vi "Simple TCP 채팅- Server.vi"() -> ()   [LabVIEW 2018]
doc: "Demonstrates how to set up a basic TCP connection, send data to the specified port once a connection has been established, and terminate the connection once the data has been sent. This VI is designed to stop if the TCP connection is terminated. The data sent in this example is an array of random numbers."
panel:
  out "서버에서 받은 문자열":string
  in  "보낼 메세지":string
  in  "Client Closed":string="The client VI closed the connection."
  in  "Stop":bool
  # "Overview: Demonstrates the use of the TCP functions to initialize a TCP server that can send data to a client VI.\nInstructions:\n1. Run the VI.\n2. Open Simple TCP - Client.vi and follow the instructions on its front panel. Note that if you wait longer than 30 seconds to do this after running this VI, it will time out.\n3. Click Stop to stop the VI. Note that if you stop the client VI, this VI will stop automatically."
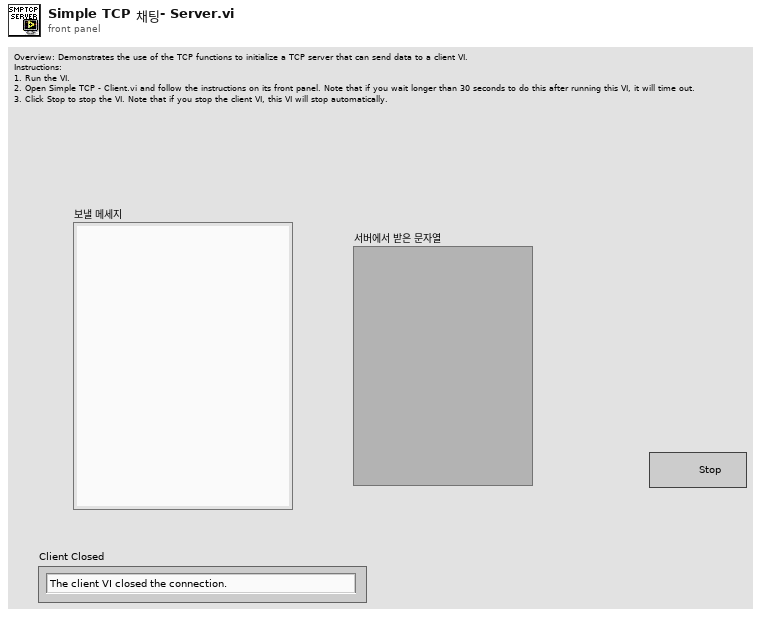
[diagram p1: front panel]
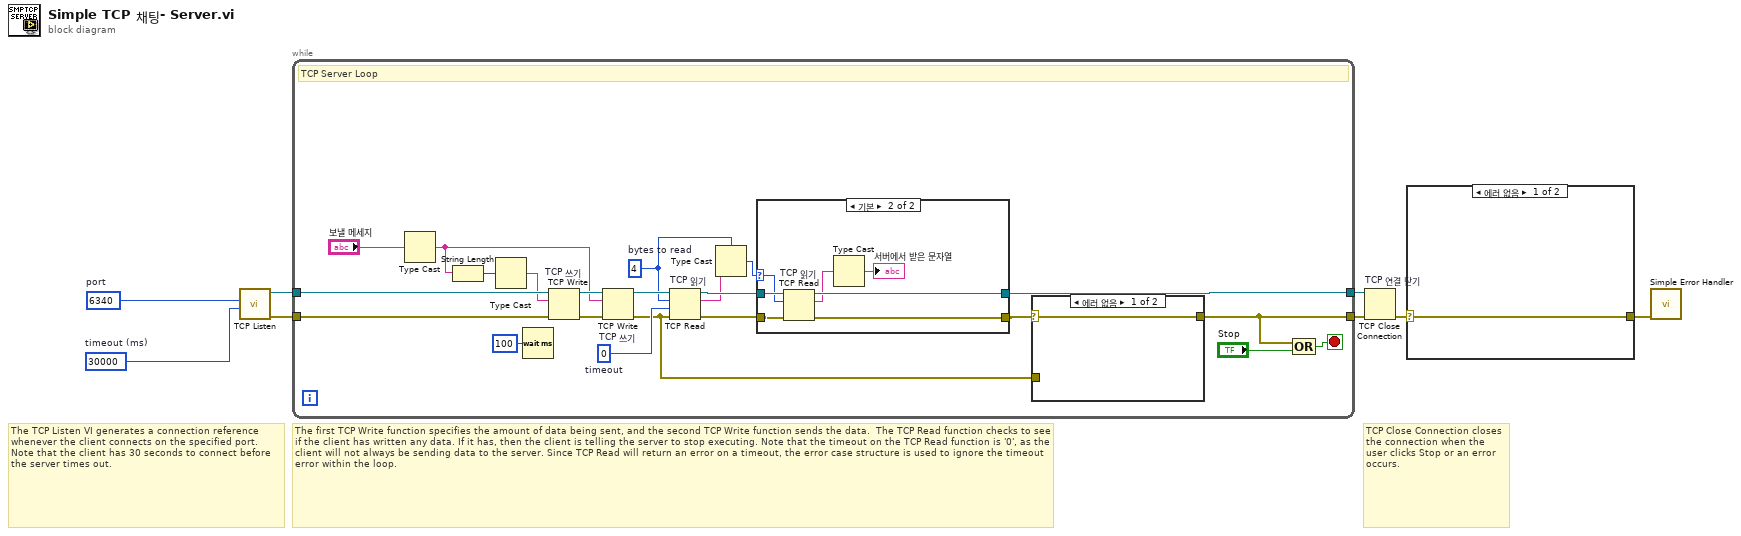
[diagram p0: block diagram]
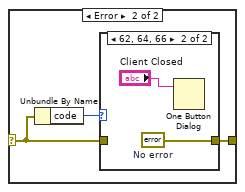
[diagram p2: hidden frame]
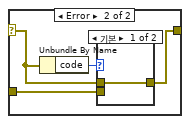
[diagram p5: hidden frame]
diagram:
  w1 = u16 6340  # port
  w2 = 30000  # timeout (ms)
  # "TCP Close Connection closes the connection when the user clicks Stop or an error occurs."
  # "The TCP Listen VI generates a connection reference whenever the client connects on the specified port. Note that the client has 30 seconds to connect before the server times out."
  # "The first TCP Write function specifies the amount of data being sent, and the second TCP Write function sends the data.  The TCP Read function checks to see if the client has written any data. If it has, then the client is telling the server to stop executing. Note that the timeout on the TCP Read function is '0', as the client will not always be sending data to the server. Since TCP Read will return an error on a timeout, the error case structure is used to ignore the timeout error within the loop."
  n1 = call <vilib>:"TCP Listen.vi"("timeout ms (wait forever: -1)"=w2, "port"=w1) -> ("error out"=w3:errorcluster, "connection ID"=w4:refnum<k5>)  [unwired: 5 in, 3 out]
  n2 = while {
    tunnel: [w18] -> w7
    tunnel: [w14] -> w8
    tunnel: w4 -> [w30]
    tunnel: w3 -> [w22]
    stop <- w23 stop-if-true
    w19 = 0  # timeout
    w11 = 4  # bytes to read
    # "TCP Server Loop"
    n3 = Type Cast(x="보낼 메세지") -> (*(type *) &x=w25:string)  [unwired: 1 out]
    n4 = String Length(string=w25) -> (length=w27:i32)
    n5 = Type Cast(x=w27) -> (*(type *) &x=w26:string)  [unwired: 1 out]
    n6 = Wait (ms)(milliseconds to wait=u32 100) -> ()  [unwired: 1 out]
    n7 = TCP Write "TCP 쓰기"(connection ID=w30, data in=w26, error in (no error)=w22) -> (connection ID out=w29:refnum<k5>, error out=w28:errorcluster)  [unwired: 2 out]
    n8 = TCP Write "TCP 쓰기"(connection ID=w29, data in=w25, error in (no error)=w28) -> (connection ID out=w20:refnum<k5>, error out=w17:errorcluster)  [unwired: 2 out]
    n9 = TCP Read "TCP 읽기"(connection ID=w20, bytes to read=w11, error in (no error)=w17, 9:w19) -> (connection ID out=w15:refnum<k5>, data out=w10:string, error out=w13:errorcluster)  [unwired: 1 out]
    n10 = Type Cast(type=w11, x=w10) -> (*(type *) &x=w9:i32)
    n11 = case shown="기본" w9 {
      selector: w9 -> [_ w34]
      tunnel: w15 -> [w32 w39]
      tunnel: w13 -> [w31 w38]
      tunnel: [w32 w37] -> w14
      tunnel: [w31 w36] -> w12
      frame ..0 {
        # "The server has not written any data"
      }
      frame Default {
        n12 = TCP Read "TCP 읽기"(connection ID=w39, bytes to read=w34, error in (no error)=w38) -> (connection ID out=w37:refnum<k5>, data out=w35:string, error out=w36:errorcluster)  [unwired: 2 in]
        n13 = Type Cast(x=w35) -> (*(type *) &x=→"서버에서 받은 문자열":string)  [unwired: 1 in]
      }
    }
    n14 = case shown="에러 없음" w12 {
      selector: w12 -> [w40 w43]
      tunnel: [w40 w41] -> w18
      tunnel: w17 -> [_ w42]
      frame No Error {
      }
      frame Error {
        n15 = Unbundle By Name(w43) -> ("code"=w44:i32)
        n16 = case shown="기본" w44 {
          tunnel: w43 -> [w45 _]
          tunnel: w42 -> [_ w46]
          tunnel: [w45 w46] -> w41
          frame Default {
          }
          frame 56 {
          }
        }
      }
    }
    n17 = Compound Arithmetic op=OR(w18, "Stop") -> (w23:bool)
  }
  n18 = TCP Close Connection "TCP 연결 닫기"(connection ID=w8, error in (no error)=w7) -> (error out=w6:errorcluster)  [unwired: 2 out]
  n19 = case shown="에러 없음" w6 {
    selector: w6 -> [w47 w49]
    tunnel: [w47 w48] -> w5
    frame No Error {
    }
    frame Error {
      n20 = Unbundle By Name(w49) -> ("code"=w50:i32)
      n21 = case shown="62, 64, 66" w50 {
        tunnel: w49 -> [w51 _]
        tunnel: [w51 w53] -> w48
        frame Default {
        }
        frame 62, 64, 66 {
          w53 = errorcluster {"status"=FALSE, "code"=0, "source"=""}  # No error
          n22 = One Button Dialog(message="Client Closed") -> ()  [unwired: 1 in, 1 out]
        }
      }
    }
  }
  n23 = call <vilib>:"Simple Error Handler.vi"("error in (no error)"=w5) -> ()  [unwired: 1 in, 8 out]
